vi "Detect P Peaks.vi"(0 "Filtered ECG":waveform(dbl)(graph)) -> (1 "P-Waves Locations (s)":dbl[](array[numeric]) format="%.2p", 2 "Coordinates":cluster{dbl[], dbl[]})   [LabVIEW 2018]
uses:
  <vilib>/measure/mamon.llb/Waveform Peak Detection for 1 Chan.vi
  <vilib>/measure/NI_MAPro.lvlib
panel:
  out "2D Low":dbl[][](array[numeric]) format="%#.2g"
  out "Unique P-Waves":dbl[](array[numeric]) format="%.2p"
  out "P-waves":dbl[](array[numeric]) format="%.2p"
  out "Clean Difference":dbl[](array[numeric]) format="%.2p"
  out "Difference":dbl[](array[numeric])
  out "Lower":dbl[](array[numeric])
  out "Upper":dbl[](array[numeric])
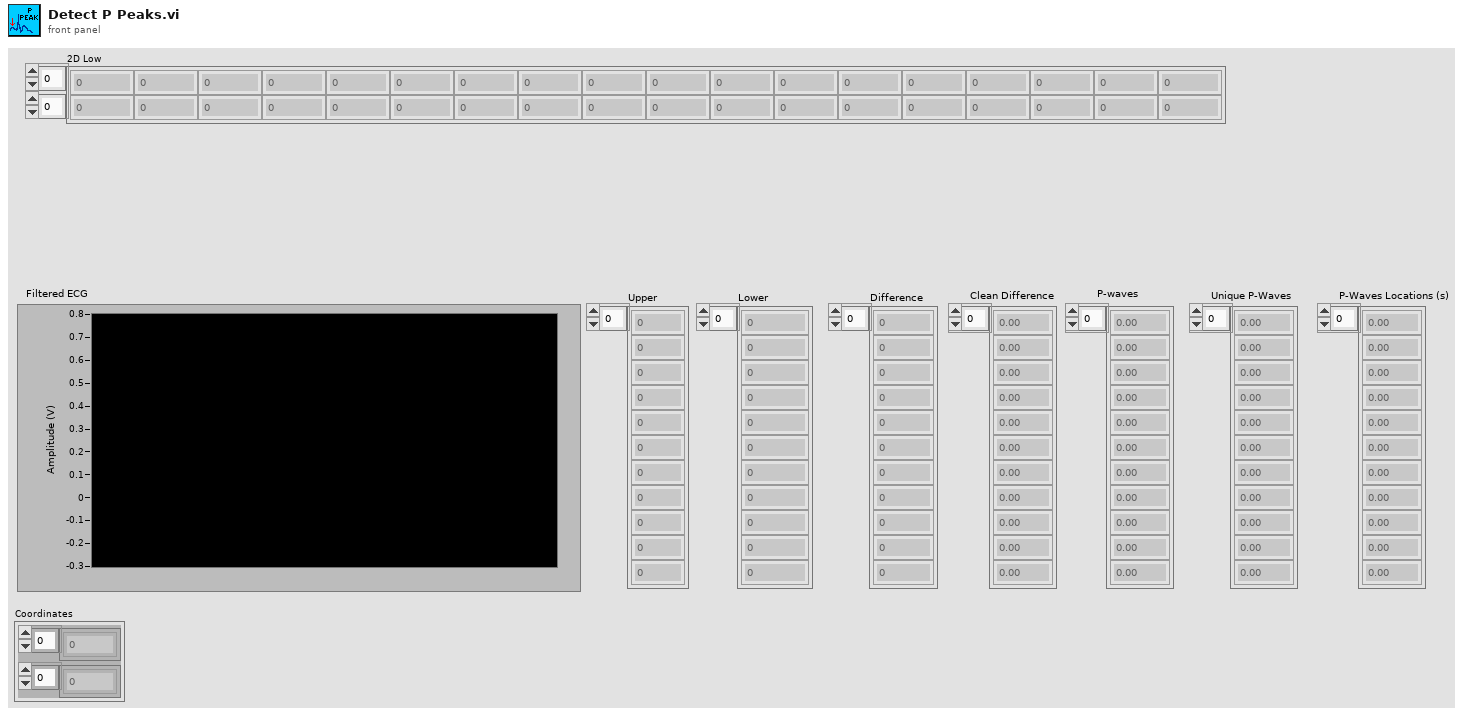
[diagram p1: front panel]
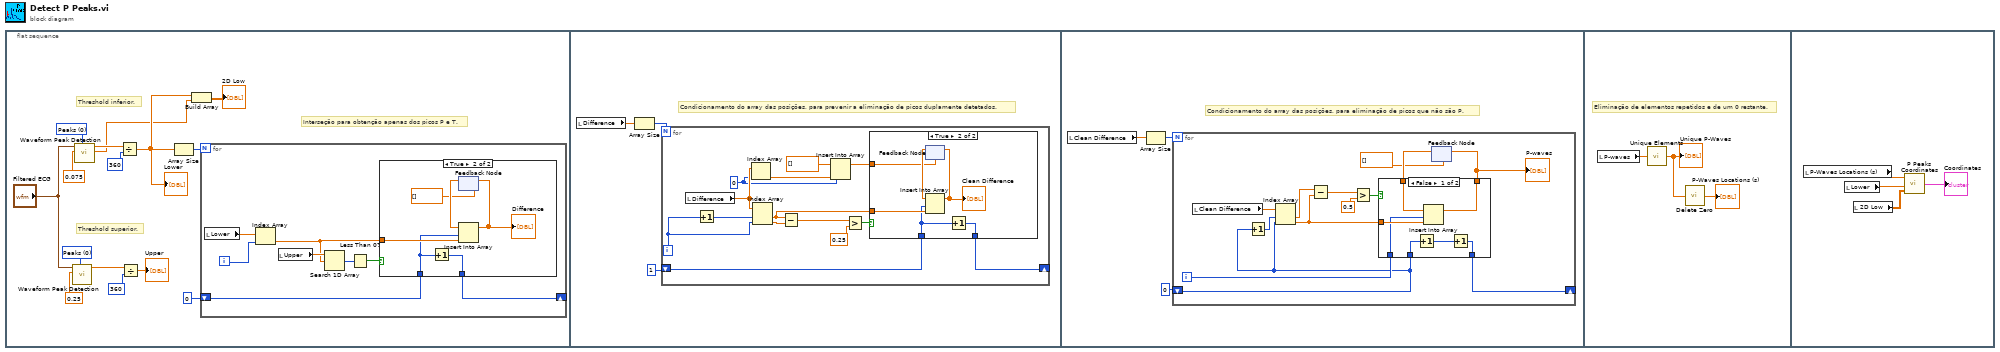
[diagram p0: block diagram]
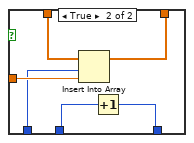
[diagram p4: hidden frame]
diagram:
  n1 = flat-sequence {
    frame #0 {
      w10 = u16 0 items=["Peaks", "Valleys"] ("peaks/valleys")
      w7 = u16 0 items=["Peaks", "Valleys"] ("peaks/valleys")
      # "Interseção para obtenção apenas dos picos P e T."
      # "Threshold inferior."
      # "Threshold superior."
      n2 = call-poly <vilib>:"Waveform Peak Detection.vi"("peaks/valleys"=w7, "threshold"=0.25 ("threshold peak"), "Signal In"="Filtered ECG") -> ("Locations"=w12:dbl[])  [unwired: 4 in, 4 out]
      n3 = call-poly <vilib>:"Waveform Peak Detection.vi"("peaks/valleys"=w10, "threshold"=0.075 ("threshold peak"), "Signal In"="Filtered ECG") -> ("Amplitudes"=w3:dbl[], "Locations"=w13:dbl[])  [unwired: 4 in, 3 out]
      n4 = Divide(x=w13, y=360 ("width")) -> (x/y=w4:dbl[])
      "Lower" <- w4
      n5 = Divide(x=w12, y=360 ("width")) -> (x/y=→"Upper":dbl[])
      n6 = Array Size(array=w4) -> (size(s)=w15:i32)
      n7 = Build Array(w4, w3) -> (→"2D Low":dbl[][])
      n8 = for {
        N: w15 -> [_]
        shift-right: [w16] -> _
        shift-left: 0 -> [w17]
        i -> [w21]
        n9 = local read "Lower"() -> (w23:dbl[])
        n10 = Index Array(array=w23, index=w21) -> (element=w19:dbl)
        n11 = local read "Upper"() -> (w22:dbl[])
        n12 = Search 1D Array(1D array=w22, element=w19) -> (index of element=w20:i32)  [unwired: 1 in]
        n13 = Less Than 0?(x=w20) -> (x < 0?=w18:bool)
        n14 = case shown="True" w18 {
          tunnel: w19 -> [_ w28]
          tunnel: w17 -> [w24 w26]
          tunnel: [w24 w25] -> w16
          frame False {
          }
          frame True {
            n15 = Increment(x=w26) -> (x+1=w25:i32)
            n16 = feedback #1(dbl[] []) -> (w30:dbl[])
            n17 = Insert Into Array(array=w30, index=w26, new element=w28) -> (w27:dbl[])
            "Difference" <- w27
            n18 = feedback-in #1(w27) -> ()
          }
        }
      }
    }
    frame #1 {
      # "Condicionamento do array das posições, para prevenir a eliminação de picos duplamente detetados."
      n19 = local read "Difference"() -> (w32:dbl[])
      n20 = Array Size(array=w32) -> (size(s)=w33:i32)
      n21 = for {
        N: w33 -> [_]
        shift-right: [w34] -> _
        shift-left: 1 -> [w35]
        i -> [w36]
        w42 = 0 ("width")
        n22 = local read "Difference"() -> (w44:dbl[])
        n23 = Increment(x=w36) -> (x+1=w37:i32)
        n24 = Index Array(array=w44, index=w42) -> (element=w43:dbl)
        n25 = Index Array(array=w44, index #1=w37, index #2=w36) -> (element #1=w38:dbl, element #2=w39:dbl)
        n26 = Subtract(x=w38, y=w39) -> (x-y=w47:dbl)
        n27 = Insert Into Array(array=dbl[] [], index=w42, new element=w43) -> (w40:dbl[])
        n28 = Greater?(x=w47, y=0.25) -> (0:w45:bool)
        n29 = case shown="True" w45 {
          tunnel: w38 -> [_ w52]
          tunnel: w40 -> [_ w51]
          tunnel: w35 -> [w48 w49]
          tunnel: [w48 w50] -> w34
          frame False {
          }
          frame True {
            n30 = feedback #2(w51) -> (w54:dbl[])
            n31 = Insert Into Array(array=w54, index=w49, new element=w52) -> (w53:dbl[])
            "Clean Difference" <- w53
            n32 = feedback-in #2(w53) -> ()
            n33 = Increment(x=w49) -> (x+1=w50:i32)
          }
        }
      }
    }
    frame #2 {
      # "Condicionamento do array das posições, para eliminação de picos que não são P."
      n34 = local read "Clean Difference"() -> (w57:dbl[])
      n35 = Array Size(array=w57) -> (size(s)=w56:i32)
      n36 = for {
        N: w56 -> [_]
        shift-right: [w58] -> _
        shift-left: 0 -> [w59]
        i -> [w60]
        n37 = local read "Clean Difference"() -> (w70:dbl[])
        n38 = Increment(x=w59) -> (x+1=w64:i32)
        n39 = Index Array(array=w70, index #1=w64, index #2=w59) -> (element #1=w69:dbl, element #2=w65:dbl)
        n40 = Subtract(x=w69, y=w65) -> (x-y=w68:dbl)
        n41 = Greater?(x=w68, y=0.5) -> (0:w66:bool)
        n42 = feedback #3(dbl[] []) -> (w63:dbl[])
        n43 = case shown="False" w66 {
          tunnel: w65 -> [w77 w83]
          tunnel: w63 -> [w76 w82]
          tunnel: [w75 w81] -> w61
          tunnel: w59 -> [w74 w80]
          tunnel: [w72 w79] -> w58
          tunnel: w60 -> [w71 w78]
          frame False {
            n44 = Increment(x=w74) -> (x+1=w73:i32)
            n45 = Insert Into Array(array=w76, index=w71, new element=w77) -> (w75:dbl[])
            n46 = Increment(x=w73) -> (x+1=w72:i32)
          }
          frame True {
            n47 = Insert Into Array(array=w82, index=w78, new element=w83) -> (w81:dbl[])
            n48 = Increment(x=w80) -> (x+1=w79:i32)
          }
        }
        "P-waves" <- w61
        n49 = feedback-in #3(w61) -> ()
      }
    }
    frame #3 {
      # "Eliminação de elementos repetidos e de um 0 restante."
      n50 = local read "P-waves"() -> (w86:dbl[])
      n51 = call "Unique Elements.vi"("P-waves"=w86) -> ("Unique P-Waves"=w85:dbl[])
      "Unique P-Waves" <- w85
      n52 = call "Delete Zero.vi"("Unique P-Waves"=w85) -> ("P-Waves Locations (s)"=→"P-Waves Locations (s)":dbl[])
    }
    frame #4 {
      n53 = local read "P-Waves Locations (s)"() -> (w90:dbl[])
      n54 = local read "Lower"() -> (w89:dbl[])
      n55 = local read "2D Low"() -> (w88:dbl[][])
      n56 = call "P Peaks Coordinates.vi"("2D Low + Amp"=w88, "Lower"=w89, "P-Wave Location (s)"=w90) -> ("P Peaks Coords"=→"Coordinates":cluster{dbl[], dbl[]})
    }
  }
